vi "Activity Light - Init.vi"(8 "error in":errorcluster, 10 "Boolean LED":refnum<vi>, 11 "Name":string="Activity Light") -> (0 "error out":errorcluster, 2 "VI Refnum":refnum<vi>)   [LabVIEW 2024, in "EQMF.lvlib" / "Status Utils.lvlib"]
uses:
  Status Utils.lvlib
  Activity Light - Core.vi
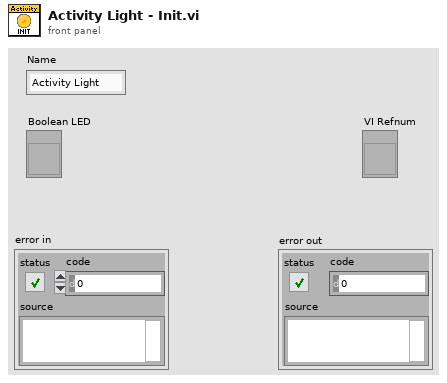
[diagram p1: front panel]
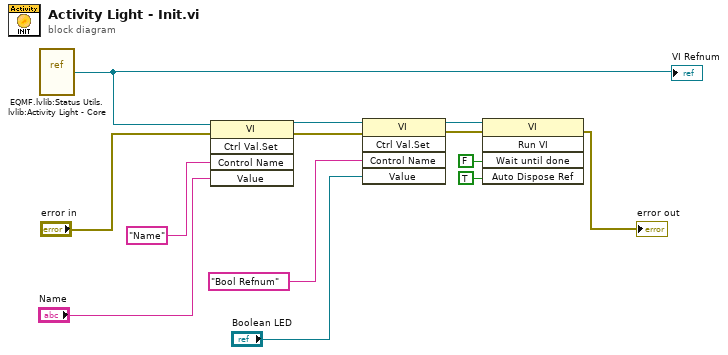
[diagram p0: block diagram]
diagram:
  n1 = vi-ref "EQMF.lvlib:Status Utils.lvlib:Activity Light - Core.vi"() -> (w4:refnum<vi>)
  "VI Refnum" <- w4
  n2 = invoke class="VI" method="Ctrl Val.Set"(reference=w4, error in="error in", "Control Name"="Name", "Value"="Name") -> (reference out=w6:refnum<vi>, error out=w5:errorcluster)  [unwired: 1 in, 3 out]
  n3 = invoke class="VI" method="Ctrl Val.Set"(reference=w6, error in=w5, "Control Name"="Bool Refnum", "Value"="Boolean LED") -> (reference out=w11:refnum<vi>, error out=w7:errorcluster)  [unwired: 1 in, 3 out]
  n4 = invoke class="VI" method="Run VI"(reference=w11, error in=w7, "Wait until done"=FALSE ("Wait Until Done"), "Auto Dispose Ref"=TRUE ("Auto Dispose Reference")) -> (error out=→"error out":errorcluster)  [unwired: 1 in, 4 out]
